vi "RNN.vi"() -> ()   [LabVIEW 2014]
panel:
  in  "Parent_Directory":path=path "C:/misc/LabVIEW/FILES"
  in  "seq_final":path=path "C:/misc/LabVIEW/FILES"
  in  "seq_inc":path=path "C:/misc/LabVIEW/FILES"
  in  "seq_init":path=path "C:/misc/LabVIEW/FILES"
  in  "states_final":path=path "C:/misc/LabVIEW/FILES"
  in  "states_inc":path=path "C:/misc/LabVIEW/FILES"
  in  "states_init":path=path "C:/misc/LabVIEW/FILES"
  in  "params_final":path=path "C:/misc/LabVIEW/FILES"
  in  "params_inc":path=path "C:/misc/LabVIEW/FILES"
  in  "params_init":path=path "C:/misc/LabVIEW/FILES"
  out "Params Saved ?":bool
  out "output_paths":path[](array[path])=[path "C:/misc/LabVIEW/FILES/Wxh_2019080217313581.psv", path "C:/misc/LabVIEW/FILES/Whh_2019080217313581.psv", path "C:/misc/LabVIEW/FILES/bh_2019080217313581.psv", path "C:/misc/LabVIEW/FILES/Why_2019080217313581.psv", path "C:/misc/LabVIEW/FILES/by_2019080217313581.psv"]
  in  "Child_Directory":path=path "C:/misc/LabVIEW/FILES"
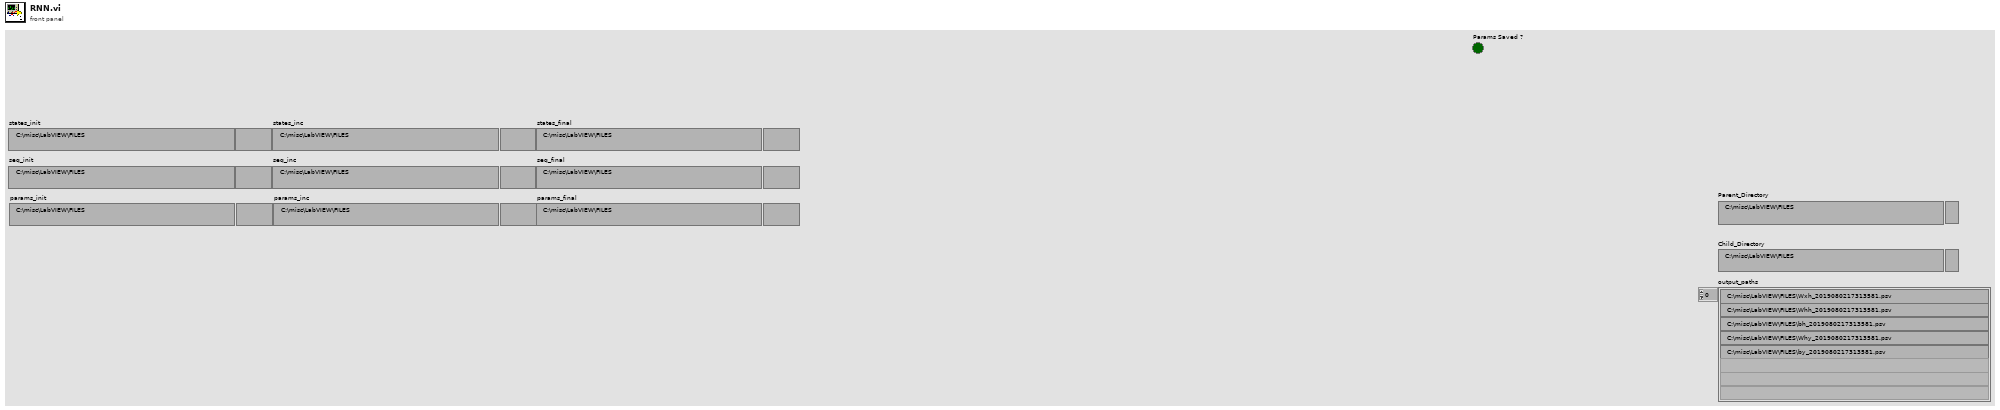
[diagram p1: front panel]
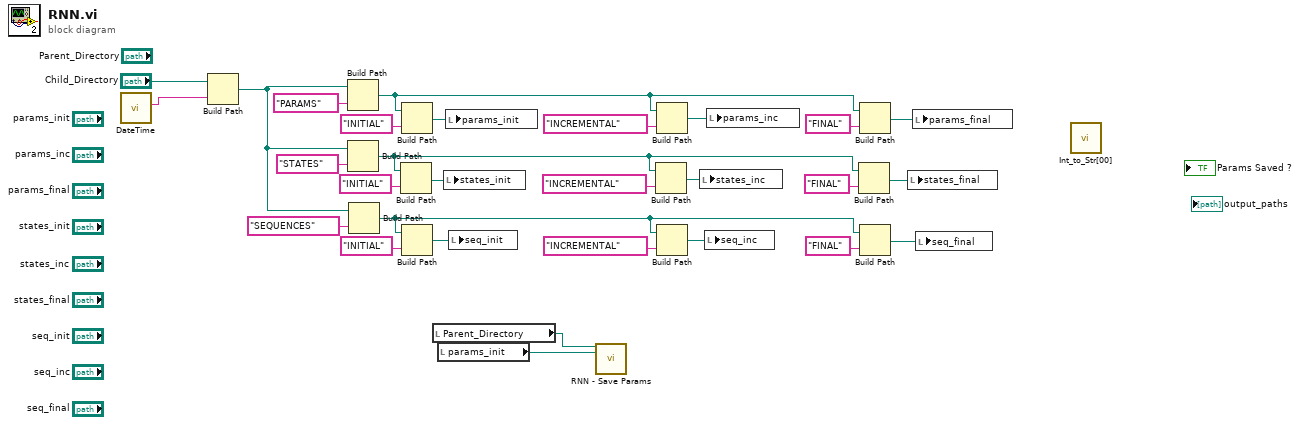
[diagram p0: block diagram]
diagram:
  n1 = call "DateTime.vi"() -> ("timestamp"=w13:string)  [unwired: 11 in]
  n2 = Build Path(base path="Child_Directory", name or relative path=w13) -> (appended path=w12:path)
  n3 = Build Path(base path=w12, name or relative path="PARAMS") -> (appended path=w24:path)
  n4 = Build Path(base path=w12, name or relative path="STATES") -> (appended path=w20:path)
  n5 = Build Path(base path=w12, name or relative path="SEQUENCES") -> (appended path=w15:path)
  n6 = Build Path(base path=w20, name or relative path="INITIAL") -> (appended path=w6:path)
  n7 = Build Path(base path=w24, name or relative path="INITIAL") -> (appended path=w11:path)
  n8 = Build Path(base path=w15, name or relative path="INITIAL") -> (appended path=w3:path)
  n9 = local read "Parent_Directory"() -> (w2:path)
  n10 = local read "params_init"() -> (w1:path)
  n11 = local write "states_init"(w6) -> ()
  n12 = local write "params_init"(w11) -> ()
  n13 = local write "seq_init"(w3) -> ()
  n14 = call "RNN - Save Params.vi"("Parent Directory"=w2, "Child Directory"=w1) -> ()  [unwired: 16 in, 2 out]
  n15 = Build Path(base path=w20, name or relative path="INCREMENTAL") -> (appended path=w7:path)
  n16 = Build Path(base path=w24, name or relative path="INCREMENTAL") -> (appended path=w10:path)
  n17 = Build Path(base path=w15, name or relative path="INCREMENTAL") -> (appended path=w4:path)
  n18 = local write "states_inc"(w7) -> ()
  n19 = local write "seq_inc"(w4) -> ()
  n20 = local write "params_inc"(w10) -> ()
  n21 = Build Path(base path=w20, name or relative path="FINAL") -> (appended path=w8:path)
  n22 = Build Path(base path=w24, name or relative path="FINAL") -> (appended path=w9:path)
  n23 = Build Path(base path=w15, name or relative path="FINAL") -> (appended path=w5:path)
  n24 = local write "states_final"(w8) -> ()
  n25 = local write "params_final"(w9) -> ()
  n26 = local write "seq_final"(w5) -> ()
  n27 = call "Int_to_Str[00].vi"() -> ()  [unwired: 19 in, 1 out]
